vi "1,3A PWM-MotorControl and VBattSense FPGA.vi"() -> ()   [LabVIEW 2011]
doc: "FPGA VI for motor control and VBAttery Sensing.\n\nMotor Control:\nBoth servos are linked to seperate I/O terminals. The Generate Digital Pulse VI inouts the PUlsewidth in us (outputted by the 1.3A PWM Motor Control VI) and creates corresponding pulses on the pins. The clock timer determines the PWM cycle time."
uses:
  SPI_State.ctl
  <vilib>/Platform/TimedLoop/XDataNode/timing_clust.ctl
  <vilib>/Platform/TimedLoop/XDataNode/nitl_modes.ctl
  <vilib>/Platform/TimedLoop/XDataNode/wakeup.ctl
  <vilib>/rvi/eio/common/nirviEmuTemplateMethod_errors.vi
  <vilib>/robotics/Utilities/FPGA Utilities/Generate Digital Pulse (uSec).vi
  <vilib>/eio/EIONode/EIONode.xnode
  <vilib>/Platform/TimedLoop/XDataNode/XDataNode.xnode
  <vilib>/robotics/Utilities/FPGA Utilities/NI_Robotics_FPGA Utilities.lvlib
  <vilib>/Platform/TimedLoop/XDataNode/XDNodeRunTimeDep.lvlib
panel:
  in  "Tab Control":enum32{"PWM", "Manual"}(tab)
  in  "Winch Duty (uSec)":u32
  in  "Rudder Duty (uSec)":u32
  in  "Rudder":bool
  in  "Winch":bool
  out "VBatt Sense Iterations":i32
  out "Averaged bitstring":bool[](array[boolean])
  in  "VBatt samples to average":u16=1500
  out "vBatt ADC bits":u16
  in  "stop VBatt Sense":bool
  in  "stop PWM":bool
  # "IF YOU HAVE TROUBLE RUNNING THIS: \ncheck if you're running it on FPGA target"
  # "Winch"
  # "Rudder"
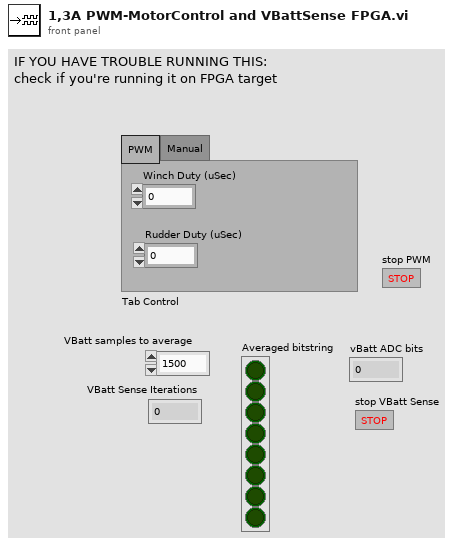
[diagram p1: front panel]
types:
  T1 = typedef "SPI_State.ctl" = enum8{"Start Read", "Transition", "Wait Cycles", "End Read"}
  T2 = typedef "XDNodeRunTimeDep.lvlib/timing_clust.ctl" = cluster{"Expected End [f-1]":u64, "Actual End [f-1]":u64, "Finished Late? [f-1]":bool, "Expected End [i-1]":u64, "Actual End [i-1]":u64, "Finished Late? [i-1]":bool, "Expected Start [i]":u64, "Actual Start [i]":u64, "Expected Start [f]":u64, "Actual Start [f]":u64, "Source Name":string, "Structure Name":string, "Period":i64, "Deadline":i64, "Offset":i64, "Start":i64, "Priority":i32, "Timeout":i32, "Mode":T3, "Wakeup Reason":T4, "Error":errorcluster, "Source Type":string, "Secondary Source Type":string, "Global End Time":u64, "Global Start Time":u64, "Frame Duration":u64, "Iteration Duration":u64, "Assigned CPU":i32, "I/O Scan Engine Mode":u32}
  T3 = typedef "XDNodeRunTimeDep.lvlib/nitl_modes.ctl" = enum32{"No Change", "Process missed periods, maintain original phase", "Discard missed periods, maintain original phase", "Process missed periods, ignore original phase", "Discard missed periods, ignore original phase"}
  T4 = typedef "XDNodeRunTimeDep.lvlib/wakeup.ctl" = enum32{"Normal", "Aborted", "Asynchronous wakeup", "Timing source error", "Timed loop error", "Timeout"}
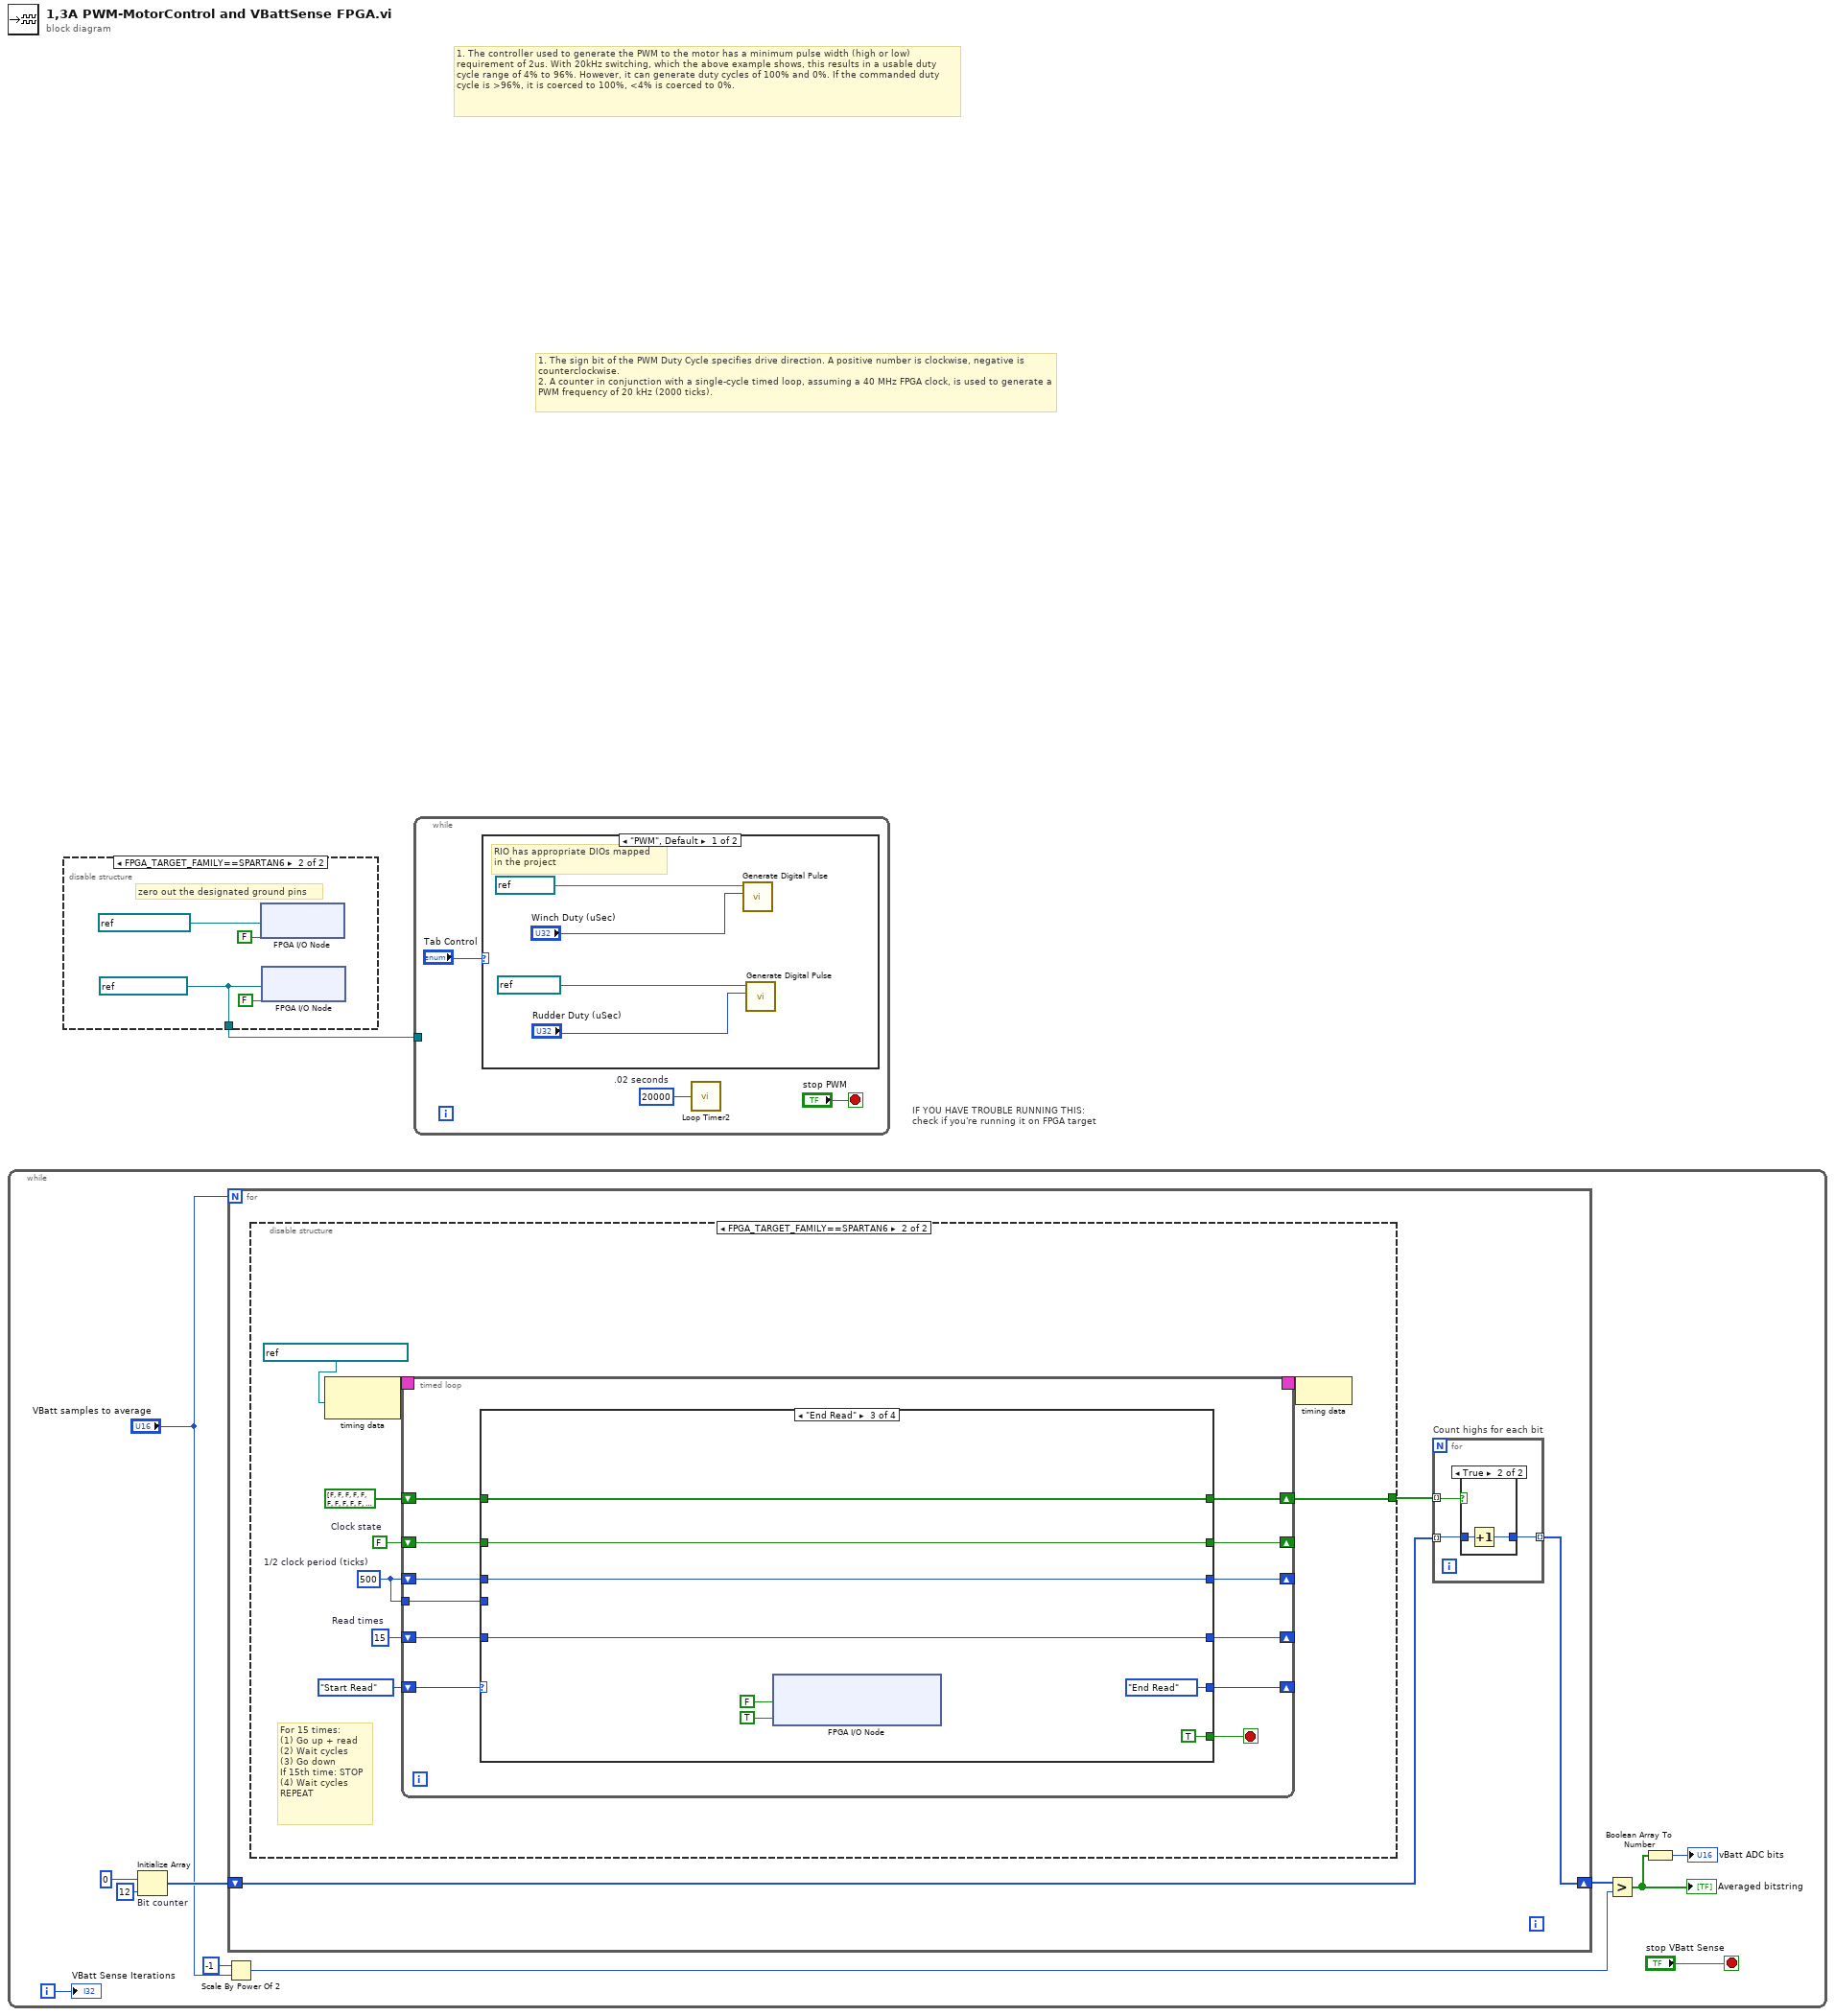
[diagram p0: block diagram]
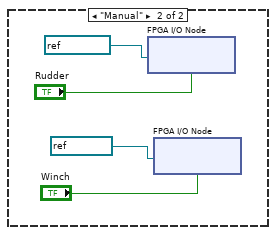
[diagram p2: hidden frame]
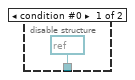
[diagram p3: hidden frame]
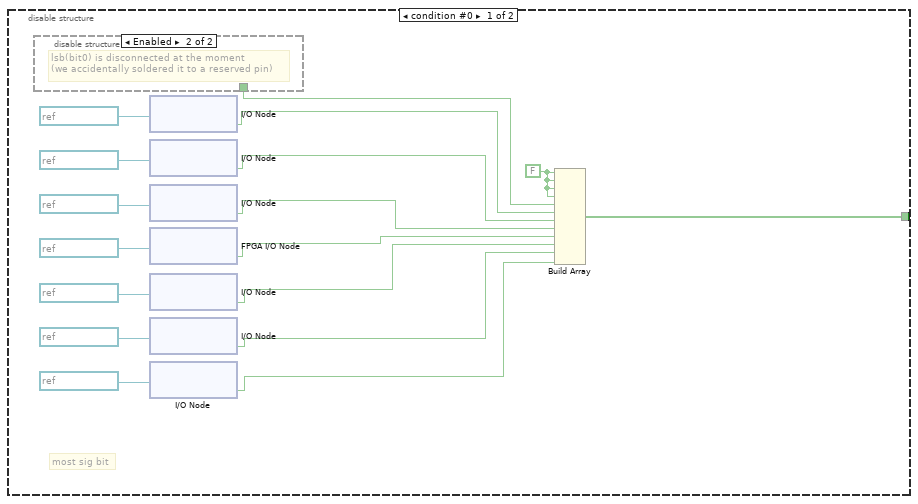
[diagram p4: hidden frame]
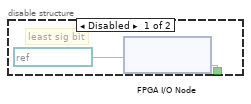
[diagram p5: hidden frame]
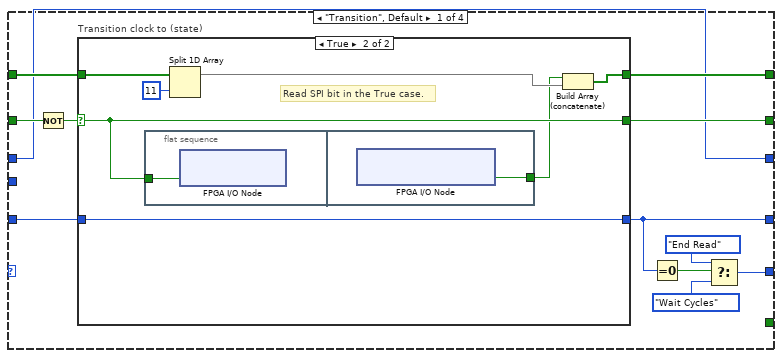
[diagram p6: hidden frame]
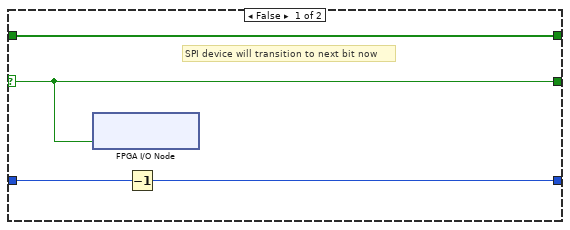
[diagram p7: hidden frame]
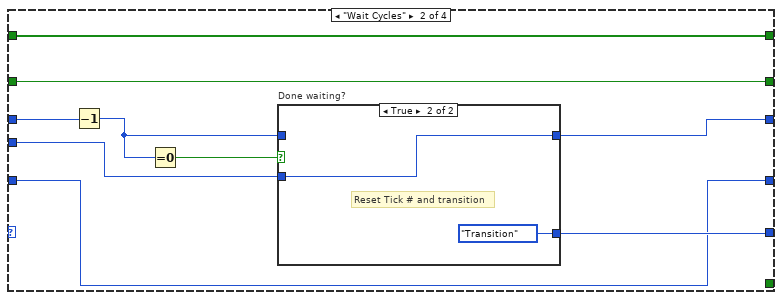
[diagram p8: hidden frame]
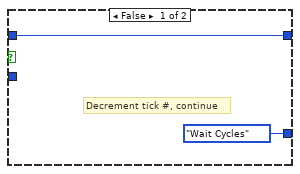
[diagram p9: hidden frame]
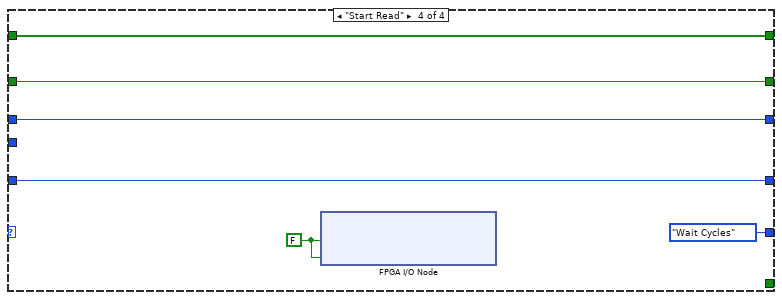
[diagram p10: hidden frame]
diagram:
  # "IF YOU HAVE TROUBLE RUNNING THIS: \ncheck if you're running it on FPGA target"
  # "1. The sign bit of the PWM Duty Cycle specifies drive direction. A positive number is clockwise, negative is counterclockwise.\n2. A counter in conjunction with a single-cycle timed loop, assuming a 40 MHz FPGA clock, is used to generate a PWM frequency of 20 kHz (2000 ticks)."
  # "1. The controller used to generate the PWM to the motor has a minimum pulse width (high or low) requirement of 2us. With 20kHz switching, which the above example shows, this results in a usable duty cycle range of 4% to 96%. However, it can generate duty cycles of 100% and 0%. If the commanded duty cycle is >96%, it is coerced to 100%, <4% is coerced to 0%."
  n1 = while {
    i -> [w9]
    stop <- "stop VBatt Sense" stop-if-true
    n2 = Initialize Array "Bit counter"(u16 0 ("VBatt Samples to read/2 2"), 12 ("dimension size")) -> (w6:u16[])
    n3 = Scale By Power Of 2(n=-1, x="VBatt samples to average") -> (x*2^n=w5:u16)
    n4 = for {
      N: "VBatt samples to average" -> [_]
      shift-right: [w13] -> w12
      shift-left: w6 -> [w15]
      n5 = disable-structure shown="FPGA_TARGET_FAMILY==SPARTAN6" {
        disable-tunnel: [w17 w38] -> w14
        frame condition #0 {
          w16 = FALSE ("element")
          # "most sig bit"
          n6 = disable-structure shown="Enabled" {
            disable-tunnel: [w33 _] -> w18
            frame Disabled {
              # "least sig bit"
              n7 = xnode "FPGA I/O Node"("FPGA I/O In"=refnum<k21> "VBatt bit0") -> ("I/O Item"=w33:bool)  [unwired: 1 out]
            }
            frame Enabled {
              # "lsb(bit0) is disconnected at the moment\n(we accidentally soldered it to a reserved pin)"
            }
          }
          n8 = xnode "I/O Node"("FPGA I/O In"=refnum<k21> "VBatt bit1") -> ("I/O Item"=w26:bool)  [unwired: 1 out]
          n9 = xnode "I/O Node"("FPGA I/O In"=refnum<k21> "VBatt bit2") -> ("I/O Item"=w27:bool)  [unwired: 1 out]
          n10 = xnode "I/O Node"("FPGA I/O In"=refnum<k21> "VBatt bit3") -> ("I/O Item"=w28:bool)  [unwired: 1 out]
          n11 = xnode "FPGA I/O Node"("FPGA I/O In"=refnum<k21> "VBatt bit4") -> ("I/O Item"=w29:bool)  [unwired: 1 out]
          n12 = xnode "I/O Node"("FPGA I/O In"=refnum<k21> "VBatt bit5") -> ("I/O Item"=w30:bool)  [unwired: 1 out]
          n13 = xnode "I/O Node"("FPGA I/O In"=refnum<k21> "VBatt bit6") -> ("I/O Item"=w31:bool)  [unwired: 1 out]
          n14 = xnode "I/O Node"("FPGA I/O In"=refnum<k21> "VBatt bit7") -> ("I/O Item"=w32:bool)  [unwired: 1 out]
          n15 = Build Array(w16, w16, w16, w16, w18, w26, w27, w28, w29, w30, w31, w32) -> (w17:bool[])
        }
        frame condition #1 (active) {
          w39 = u32 500  # 1/2 clock period (ticks)
          w40 = FALSE  # Clock state
          w41 = u8 15  # Read times
          # "For 15 times:\n(1) Go up + read\n(2) Wait cycles\n(3) Go down\nIf 15th time: STOP\n(4) Wait cycles\nREPEAT"
          n16 = node-c288(refnum<k21> "40 MHz Onboard Clock" ("Source Name")) -> (w37:T2)
          n17 = timed-loop {
            shift-right: [w48] -> _
            shift-left: SPI_State."Start Read" ("Action") -> [w55]
            shift-right: [w51] -> w38
            shift-left: bool[] [FALSE, FALSE, FALSE, FALSE, FALSE, FALSE, FALSE, FALSE, FALSE, FALSE, FALSE, FALSE] ("Battery Voltage") -> [w52]
            shift-right: [w53] -> _
            shift-left: w40 -> [w54]
            tunnel: w39 -> [w46]
            shift-right: [w45] -> _
            shift-left: w39 -> [w47]
            shift-right: [w49] -> _
            shift-left: w41 -> [w50]
            timing: w37 -> [_]
            timing-out: [_] -> w36
            stop <- w44 stop-if-true
            n18 = case shown="\"End Read\"" w55 {
              tunnel: w54 -> [w67 w89 w97 w105]
              tunnel: [w66 w89 w97 w105] -> w53
              tunnel: w52 -> [w64 w88 w96 w106]
              tunnel: [w63 w88 w96 w106] -> w51
              tunnel: w50 -> [w62 w81 w100 w103]
              tunnel: [w60 w81 w100 w103] -> w49
              tunnel: [w58 w84 SPI_State."End Read" ("Action") SPI_State."Wait Cycles" ("Action")] -> w48
              tunnel: w47 -> [w61 w87 w98 w104]
              tunnel: w46 -> [_ w82 _ _]
              tunnel: [w61 w83 w98 w104] -> w45
              tunnel: [_ _ TRUE _] -> w44
              frame "Transition", Default {
                n19 = Not(x=w67) -> (.not. x?=w65:bool)
                n20 = case "Transition clock to (state)" shown="True" w65 {
                  selector: w65 -> [w71 w78]
                  tunnel: [w71 w78] -> w66
                  tunnel: w64 -> [w68 w77]
                  tunnel: [w68 w75] -> w63
                  tunnel: w62 -> [w70 w74]
                  tunnel: [w69 w74] -> w60
                  frame False {
                    # "SPI device will transition to next bit now"
                    n21 = xnode "FPGA I/O Node"("VBatt_Clock"=w71) -> ()  [unwired: 1 in, 1 out]
                    n22 = Decrement(x=w70) -> (x-1=w69:u8)
                  }
                  frame True {
                    # "Read SPI bit in the True case."
                    n23 = flat-sequence {
                      tunnel: w78 -> [w79]
                      tunnel: [w80] -> w72
                      frame #0 {
                        n24 = xnode "FPGA I/O Node"("VBatt_Clock"=w79) -> ()  [unwired: 1 in, 1 out]
                      }
                      frame #1 {
                        n25 = xnode "FPGA I/O Node"() -> ("VBatt_DigitalInput"=w80:bool)  [unwired: 1 in, 1 out]
                      }
                    }
                    n26 = Split 1D Array(array=w77, index=11) -> (first subarray=w73:bool[])  [unwired: 1 out]
                    n27 = Build Array (concatenate)(w72, w73) -> (w75:bool[])
                  }
                }
                n28 = Equal To 0?(x=w60) -> (x = 0?=w59:bool)
                n29 = Select(t=SPI_State."End Read" ("Action"), s=w59, f=SPI_State."Wait Cycles" ("Action")) -> (s? t:f=w58:T1)
              }
              frame "Wait Cycles" {
                n30 = Decrement(x=w87) -> (x-1=w85:u32)
                n31 = Equal To 0?(x=w85) -> (x = 0?=w86:bool)
                n32 = case "Done waiting?" shown="True" w86 {
                  tunnel: w85 -> [w90 _]
                  tunnel: [SPI_State."Wait Cycles" ("Action") SPI_State."Transition" ("Action")] -> w84
                  tunnel: [w90 w92] -> w83
                  tunnel: w82 -> [_ w92]
                  frame False {
                    # "Decrement tick #, continue"
                  }
                  frame True {
                    # "Reset Tick # and transition"
                  }
                }
              }
              frame "End Read" {
                n33 = xnode "FPGA I/O Node"("VBatt_Clock"=FALSE ("VBatt_ChipSelectInverted"), "VBatt_ChipSelectInverted"=TRUE) -> ()  [unwired: 2 in, 2 out]
              }
              frame "Start Read" {
                w107 = FALSE ("VBatt_ChipSelectInverted")
                n34 = xnode "FPGA I/O Node"("VBatt_Clock"=w107, "VBatt_ChipSelectInverted"=w107) -> ()  [unwired: 2 in, 2 out]
              }
            }
          }
          n35 = node-c288(w36) -> ()
        }
      }
      n36 = for "Count highs for each bit" {
        tunnel: w14 -> [w114] mode=indexing
        tunnel: w15 -> [w113] mode=indexing
        tunnel: [w112] -> w13 mode=indexing
        n37 = case shown="True" w114 {
          tunnel: w113 -> [w115 w117]
          tunnel: [w115 w116] -> w112
          frame False {
          }
          frame True {
            n38 = Increment(x=w117) -> (x+1=w116:u16)
          }
        }
      }
    }
    n39 = Greater?(x=w12, y=w5) -> (0:w11:bool[])
    "Averaged bitstring" <- w11
    n40 = Boolean Array To Number(Boolean array=w11) -> (number=→"vBatt ADC bits":u16)
    "VBatt Sense Iterations" <- w9
  }
  n41 = disable-structure shown="FPGA_TARGET_FAMILY==SPARTAN6" {
    disable-tunnel: [refnum<k21> refnum ("FPGA digital output") w119] -> w1
    frame condition #0 {
    }
    frame condition #1 (active) {
      w119 = refnum<k21> "Winch_GND" ("FPGA digital output")
      # "zero out the designated ground pins"
      n42 = xnode "FPGA I/O Node"("I/O Item"=FALSE, "FPGA I/O In"=refnum<k21> "Rudder_GND" ("FPGA digital output")) -> ()  [unwired: 1 out]
      n43 = xnode "FPGA I/O Node"("I/O Item"=FALSE, "FPGA I/O In"=w119) -> ()  [unwired: 1 out]
    }
  }
  n44 = while {
    tunnel: w1 -> [_]
    stop <- "stop PWM" stop-if-true
    w123 = u32 20000  # .02 seconds
    n45 = case shown="\"PWM\", Default" "Tab Control" {
      frame "PWM", Default {
        # "RIO has appropriate DIOs mapped\nin the project"
        n46 = call-poly <vilib>:"Generate Digital Pulse.vi"("pulse width (uSec)"="Winch Duty (uSec)", "FPGA digital output"=refnum<k21> "Winch") -> ()  [unwired: 10 in]
        n47 = call-poly <vilib>:"Generate Digital Pulse.vi"("pulse width (uSec)"="Rudder Duty (uSec)", "FPGA digital output"=refnum<k21> "Rudder") -> ()  [unwired: 10 in]
      }
      frame "Manual" {
        n48 = xnode "FPGA I/O Node"("I/O Item"="Rudder", "FPGA I/O In"=refnum<k21> "Rudder" ("FPGA digital output")) -> ()  [unwired: 1 out]
        n49 = xnode "FPGA I/O Node"("I/O Item"="Winch", "FPGA I/O In"=refnum<k21> "Winch" ("FPGA digital output")) -> ()  [unwired: 1 out]
      }
    }
    n50 = call "Loop Timer2"("Count(uSec)"=w123) -> ()  [unwired: 1 out]
  }
